vi "to_json.vi"(8 "error in":errorcluster, 11 "csv in":refnum<class "csv.lvclass">) -> (0 "error out":errorcluster, 2 "json":string, 3 "csv out":refnum<class "csv.lvclass">, 4 "Not Default":bool)   [LabVIEW 2020, in "datasources.lvlib" / "csv.lvclass"]
uses:
  csv.lvclass
  C:/code/labview-client/lv_src/Nominal Client/datasources/datasource/datasource.lvclass
  csv.lvclass/csv.ctl
  datasource/datasource.lvclass/datasource.ctl
  3f751956-4498-4abf-b7e3-c6c77908fc4b.vi
  datasource/source.get.vi
  datasource/target.get.vi
  <vilib>/JDP Science/JSONtext/Variant to JSON Text.vi
  <vilib>/JDP Science/JSONtext/support/Format JSON Object.vi
  timestampMetadata/timestampMetadata.lvclass
  nominal types/labels/labels.lvclass
  nominal types/properties/properties.lvclass
  <vilib>/JDP Science/JSONtext/LVClass Serializer/JSONtext LVClass Serializer.lvclass
  source/source.lvclass
  target/target.lvclass
  <vilib>/JDP Science/JSONtext/JSONtext.lvlib
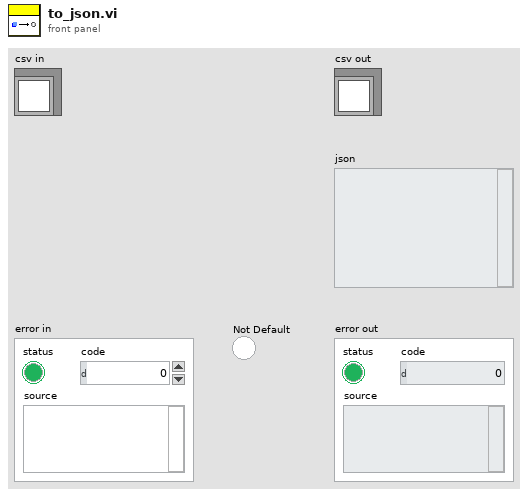
[diagram p1: front panel]
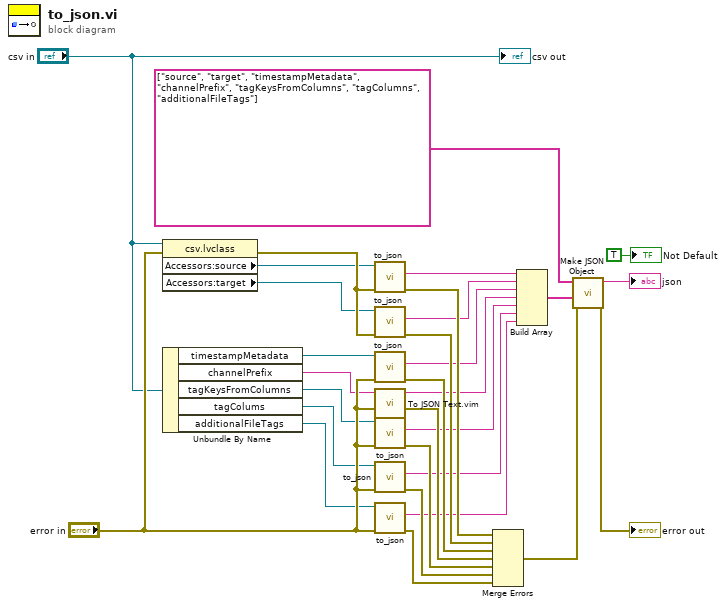
[diagram p0: block diagram]
diagram:
  n1 = property class="csv.lvclass"(reference="csv in", error in="error in") -> (error out=w30:errorcluster, "Accessors:source"=w27:refnum<class "source.lvclass">, "Accessors:target"=w28:refnum<class "target.lvclass">)  [unwired: 1 out]
  n2 = Unbundle By Name("csv in") -> ("timestampMetadata"=w26:refnum<class "timestampMetadata.lvclass">, "channelPrefix"=w22:string, "tagKeysFromColumns"=w23:refnum<class "labels.lvclass">, "tagColums"=w24:refnum<class "properties.lvclass">, "additionalFileTags"=w25:refnum<class "properties.lvclass">)
  n3 = call-dynamic "to_json.vi"("error in"=w30, "source in"=w27) -> ("error out"=w16:errorcluster, "json"=w20:string)  [unwired: 6 in, 2 out]
  n4 = call-dynamic "to_json.vi"("error in"=w30, "target in"=w28) -> ("error out"=w15:errorcluster, "json"=w7:string)  [unwired: 6 in, 2 out]
  n5 = call-dynamic "to_json.vi"("error in"="error in", "timestampMetadata in"=w26) -> ("error out"=w14:errorcluster, "json"=w6:string)  [unwired: 6 in, 2 out]
  n6 = call "To JSON Text.vim"("error in (no error)"="error in", "Anything"=w22) -> ("error out"=w13:errorcluster, "<JSON>"=w5:string)  [unwired: 8 in]
  n7 = call-dynamic "to_json.vi"("error in"="error in", "labels in"=w23) -> ("error out"=w12:errorcluster, "json"=w4:string)  [unwired: 6 in, 2 out]
  n8 = call-dynamic "to_json.vi"("error in"="error in", "properties in"=w24) -> ("error out"=w11:errorcluster, "json"=w3:string)  [unwired: 6 in, 2 out]
  n9 = call-dynamic "to_json.vi"("error in"="error in", "properties in"=w25) -> ("error out"=w10:errorcluster, "json"=w2:string)  [unwired: 6 in, 2 out]
  n10 = Merge Errors(w16, w15, w14, w13, w12, w11, w10) -> (w9:errorcluster)
  n11 = Build Array(w20, w7, w6, w5, w4, w3, w2) -> (w19:string[])
  n12 = call <vilib>:"Make JSON Object.vi"("error in (no error)"=w9, "JSON Items"=w19, "Item Names"=string[] ["source", "target", "timestampMetadata", "channelPrefix", "tagKeysFromColumns", "tagColumns", "additionalFileTags"]) -> ("error out"=→"error out":errorcluster, "<JSON>"=→"json":string)  [unwired: 7 in]
  "csv out" <- "csv in"
  "Not Default" <- TRUE ("Not Default")
